vi "createQR.vi"(8 "Error In":errorcluster, 10 "Shift":string, 11 "QR Data":T1) -> (0 "Error Out":errorcluster, 3 "QR":string)   [LabVIEW 2018]
uses:
  controls/qrData.ctl
  UI Module/src/controls/LHndRH.ctl
panel:
  in  "Production Date":string
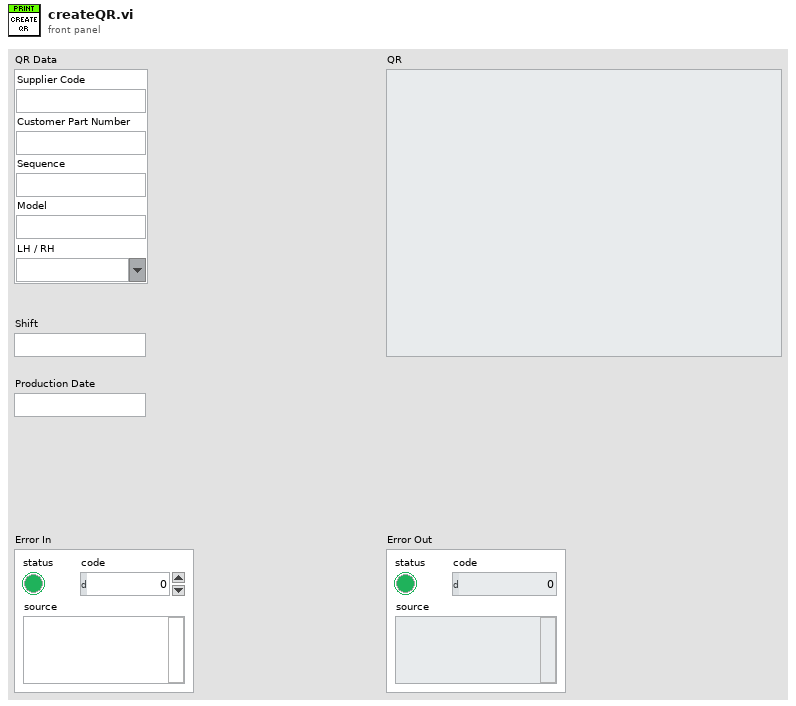
[diagram p1: front panel]
types:
  T1 = typedef "qrData.ctl" = cluster{"Supplier Code":string, "Customer Part Number":string, "Sequence":string, "Model":string, "LH / RH":T2}
  T2 = typedef "LHndRH.ctl" = string
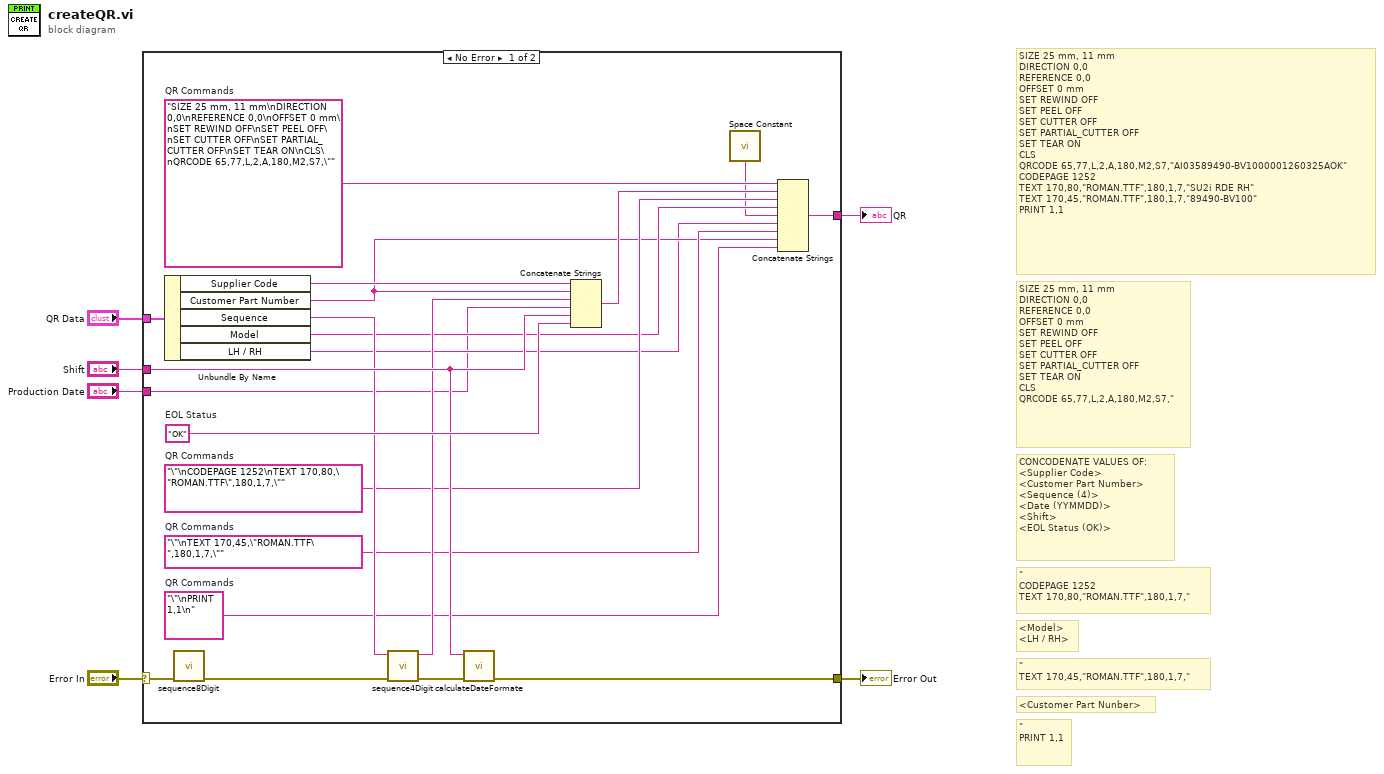
[diagram p0: block diagram]
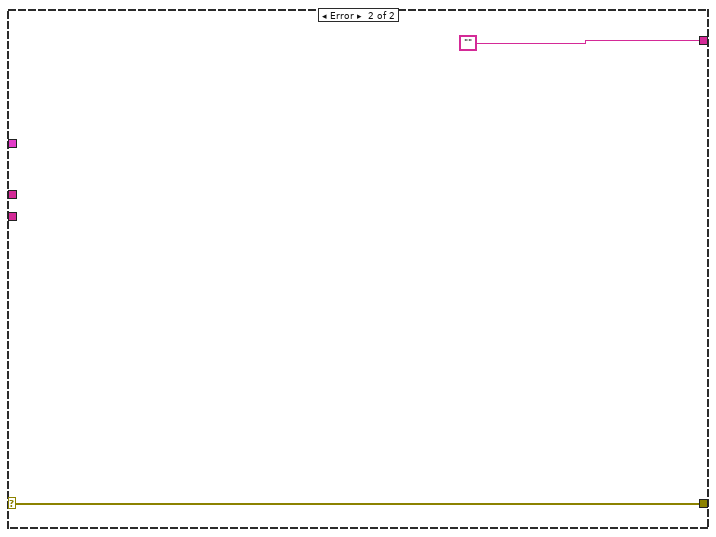
[diagram p2: hidden frame]
diagram:
  # "\"\nPRINT 1,1"
  # "<Customer Part Nunber>"
  # "\"\nTEXT 170,45,\"ROMAN.TTF\",180,1,7,\""
  # "<Model>\n<LH / RH>"
  # "\"\nCODEPAGE 1252\nTEXT 170,80,\"ROMAN.TTF\",180,1,7,\""
  # "CONCODENATE VALUES OF:\n<Supplier Code>\n<Customer Part Number>\n<Sequence (4)>\n<Date (YYMMDD)>\n<Shift>\n<EOL Status (OK)>"
  # "SIZE 25 mm, 11 mm\nDIRECTION 0,0\nREFERENCE 0,0\nOFFSET 0 mm\nSET REWIND OFF\nSET PEEL OFF\nSET CUTTER OFF\nSET PARTIAL_CUTTER OFF\nSET TEAR ON\nCLS\nQRCODE 65,77,L,2,A,180,M2,S7,\""
  # "SIZE 25 mm, 11 mm\nDIRECTION 0,0\nREFERENCE 0,0\nOFFSET 0 mm\nSET REWIND OFF\nSET PEEL OFF\nSET CUTTER OFF\nSET PARTIAL_CUTTER OFF\nSET TEAR ON\nCLS\nQRCODE 65,77,L,2,A,180,M2,S7,\"AI03589490-BV1000001260325AOK\"\nCODEPAGE 1252\nTEXT 170,80,\"ROMAN.TTF\",180,1,7,\"SU2i RDE RH\"\nTEXT 170,45,\"ROMAN.TTF\",180,1,7,\"89490-BV100\"\nPRINT 1,1"
  n1 = case shown="No Error" "Error In" {
    selector: "Error In" -> [w27 w29]
    tunnel: [w20 w29] -> w5
    tunnel: [w26 ""] -> w4
    tunnel: "QR Data" -> [w23 _]
    tunnel: "Shift" -> [w19 _]
    tunnel: "Production Date" -> [w7 _]
    frame No Error {
      w10 = "\"\nPRINT 1,1\n"  # QR Commands
      w12 = "\"\nTEXT 170,45,\"ROMAN.TTF\",180,1,7,\""  # QR Commands
      w14 = "\"\nCODEPAGE 1252\nTEXT 170,80,\"ROMAN.TTF\",180,1,7,\""  # QR Commands
      w22 = "OK"  # EOL Status
      w25 = "SIZE 25 mm, 11 mm\nDIRECTION 0,0\nREFERENCE 0,0\nOFFSET 0 mm\nSET REWIND OFF\nSET PEEL OFF\nSET CUTTER OFF\nSET PARTIAL_CUTTER OFF\nSET TEAR ON\nCLS\nQRCODE 65,77,L,2,A,180,M2,S7,\""  # QR Commands
      n2 = Unbundle By Name(w23) -> ("Supplier Code"=w24:string, "Customer Part Number"=w11:string, "Sequence"=w15:string, "Model"=w13:string, "LH / RH"=w9:T2)
      n3 = call "sequence8Digit.vi"("Error In"=w27) -> ("Error Out"=w18:errorcluster)  [unwired: 9 in, 1 out]
      n4 = call "sequence4Digit.vi"("Error In"=w18, "Trace Number In"=w15) -> ("Error Out"=w17:errorcluster, "Trace Number Out"=w16:string)  [unwired: 8 in]
      n5 = call "calculateDateFormate.vi"("Error In"=w17, "Shift"=w19) -> ("Error Out"=w20:errorcluster)  [unwired: 7 in, 2 out]
      n6 = Concatenate Strings(w24, w11, w16, w7, w19, w22) -> (w21:string)
      n7 = call <vilib>:"Space Constant.vi"() -> ("String"=w8:string)
      n8 = Concatenate Strings(w25, w21, w14, w13, w8, w9, w12, w11, w10) -> (w26:string)
    }
    frame Error {
    }
  }
  "Error Out" <- w5
  "QR" <- w4
